vi "Process_SetData.vi"(0 "ref in":T1, 1 "Data in":T2, 3 "error in":errorcluster) -> (6 "ref out":T1, 9 "error out":errorcluster)   [LabVIEW 2015]
uses:
  Control/Process_Data.ctl
  Control/Process_Mode.ctl
  Control/Process_Function.ctl
panel:
  out "Timed out":bool
  in  "ms timeout (-1)":i32=-1
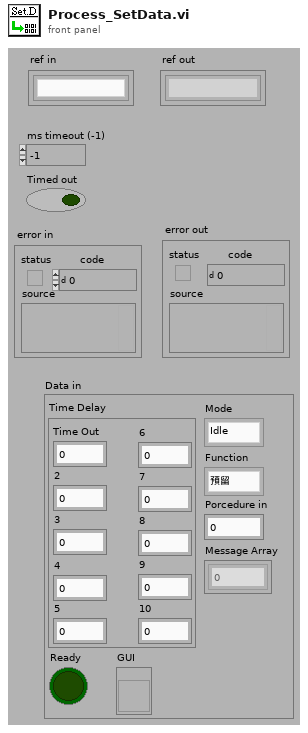
[diagram p1: front panel]
types:
  T1 = typedef "Error站_ref.ctl" = refnum<k1>
  T2 = typedef "Process_Data.ctl" = cluster{"GUI":refnum<vi>, "Ready":bool, "Mode":T3, "Function":T4, "Porcedure in":u8, "Time Delay":cluster{"Time Out":dbl, "2":dbl, "3":dbl, "4":dbl, "5":dbl, "6":dbl, "7":dbl, "8":dbl, "9":dbl, "10":dbl}, "Message Array":i32[]}
  T3 = typedef "Process_Mode.ctl" = enum8{"Idle", "Run", "Pause", "Err"}
  T4 = typedef "Process_Function.ctl" = enum8{"預留"}
  T5 = enum16{"OpenReference", "CloseReference", "Get Data", "Set Data", "Set Flag"}
  T6 = typedef "Semaphore RefNum" = refnum<k1>
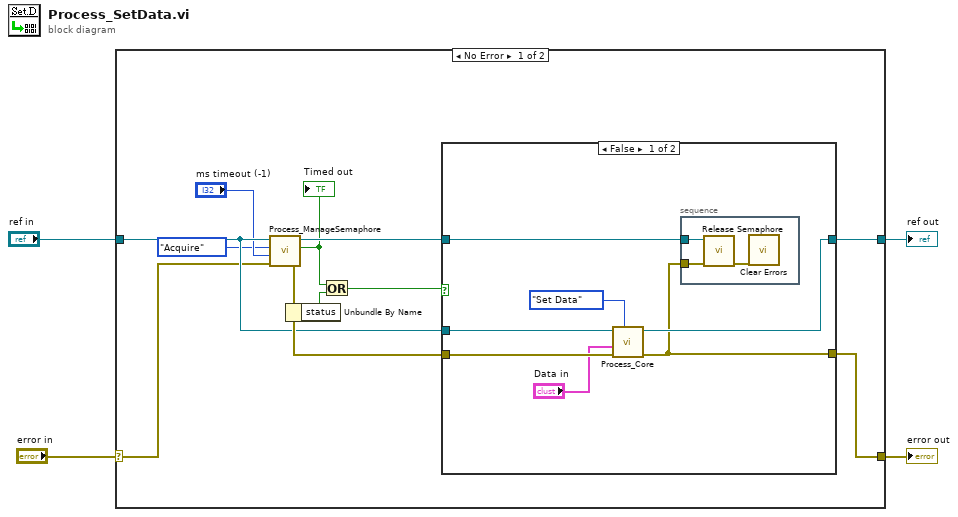
[diagram p0: block diagram]
diagram:
  n1 = case shown="No Error" "error in" {
    selector: "error in" -> [w6 w29]
    tunnel: [w10 w29] -> w3
    tunnel: "ref in" -> [w11 w28]
    tunnel: [w12 w28] -> w1
    frame No Error {
      n2 = call "Process_ManageSemaphore.vi"("error in (no error)"=w6, "ms timeout (-1)"="ms timeout (-1)", "Method (Acquire)"=enum8{"Acquire", "Destroy"}."Acquire", "ref"=w11) -> ("error out"=w15:errorcluster, "Timed out"=w7:bool, "semaphore out"=w13:T6)  [unwired: 1 in]
      "Timed out" <- w7
      n3 = Unbundle By Name(w15) -> ("status"=w8:bool)
      n4 = Or(x=w7, y=w8) -> (x .or. y?=w14:bool)
      n5 = case shown="False" w14 {
        tunnel: [w21 w26] -> w12
        tunnel: w13 -> [w22 _]
        tunnel: w15 -> [w18 w27]
        tunnel: [w20 w27] -> w10
        tunnel: w11 -> [w19 w26]
        frame False {
          n6 = call "Process_Core.vi"("Function"=T5."Set Data", "error in"=w18, "Data in"="Data in", "ref in"=w19) -> ("error out"=w20:errorcluster, "ref out"=w21:T1)  [unwired: 4 in, 2 out]
          n7 = stacked-sequence {
            tunnel: w22 -> [w25]
            tunnel: w20 -> [w23]
            frame #0 {
              n8 = call <vilib>:"Release Semaphore.vi"("error in (no error)"=w23, "semaphore"=w25) -> ("error out"=w24:errorcluster)  [unwired: 4 in, 1 out]
              n9 = call <vilib>:"Clear Errors.vi"("error in (no error)"=w24) -> ()  [unwired: 5 in, 2 out]
            }
          }
        }
        frame True {
        }
      }
    }
    frame Error {
    }
  }
  "error out" <- w3
  "ref out" <- w1
